vi "SSC Digital Apply TDR Offsets.vi"(0 "Digital SSC in":T1[](array[typedef]), 5 "Per-Instrument offsets (s)":dbl[][](array[numeric]), 11 "error in":errorcluster) -> (4 "Digital SSC out":T1[](array[typedef]), 15 "error out":errorcluster)   [LabVIEW 2020]
doc: "Applies the correction for propagation delay offsets to digital pattern instrument(s) connected to the specified pin(s) and pin group(s).\n\nUse this VI to apply TDR offsets that are stored from a past measurement or are measured by means other than the niDigital TDR VI. Also use this VI to apply correction for offsets if the apply offsets input of the niDigital TDR VI was set to False at the time of measurement."
uses:
  SSC Digital.ctl
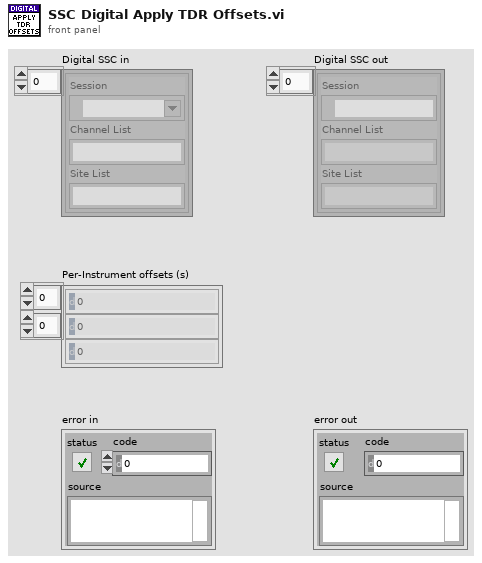
[diagram p1: front panel]
types:
  T1 = typedef "SSC Digital.ctl" = cluster{"Session":refnum<k15>, "Channel List":string, "Site List":string}
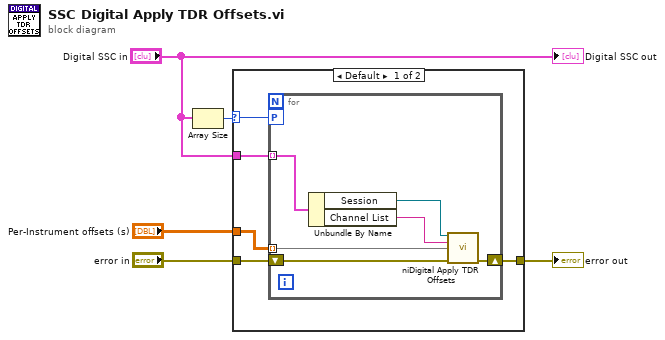
[diagram p0: block diagram]
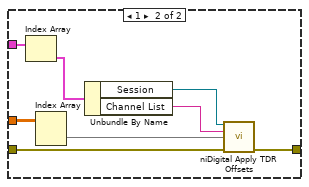
[diagram p2: hidden frame]
diagram:
  n1 = Array Size(array="Digital SSC in") -> (size(s)=w2:i32)
  n2 = case shown="Default" w2 {
    selector: w2 -> [w7 _]
    tunnel: "error in" -> [w10 w24]
    tunnel: "Per-Instrument offsets (s)" -> [w9 w23]
    tunnel: [w8 w22] -> w3
    tunnel: "Digital SSC in" -> [w6 w21]
    frame Default {
      n3 = for {
        workers-P: w7 -> [_]
        tunnel: w6 -> [w13] mode=indexing
        tunnel: w9 -> [w11] mode=indexing
        shift-right: [w15] -> w8
        shift-left: w10 -> [w16]
        n4 = Unbundle By Name(w13) -> ("Session"=w14:refnum<k15>, "Channel List"=w12:string)
        n5 = call <instrlib>:"niDigital Apply TDR Offsets.vi"("instrument handle"=w14, "channel list"=w12, "offsets (s)"=w11, "error in"=w16) -> ("error out"=w15:errorcluster)  [unwired: 10 in, 1 out]
      }
    }
    frame 1 {
      n6 = Index Array(array=w21) -> (element=w18:T1)  [unwired: 1 in]
      n7 = Index Array(array=w23) -> (element=w17:dbl[])  [unwired: 2 in]
      n8 = Unbundle By Name(w18) -> ("Session"=w20:refnum<k15>, "Channel List"=w19:string)
      n9 = call <instrlib>:"niDigital Apply TDR Offsets.vi"("instrument handle"=w20, "channel list"=w19, "offsets (s)"=w17, "error in"=w24) -> ("error out"=w22:errorcluster)  [unwired: 10 in, 1 out]
    }
  }
  "error out" <- w3
  "Digital SSC out" <- "Digital SSC in"
